vi "Pega_Tags_cluster_entrada.vi"() -> (1 "TipoVariavel":string[](array[string]), 2 "Array Tags":string[](array[string]))   [LabVIEW 2019]
uses:
  padrao_todos_os_dados_ENTRADA.ctl
  padrao_UCM.004.EEL.0300_ENTRADA.ctl
  padrao_UCM.004.EEL.0200_ENTRADA.ctl
  padrao_INTERNO.ctl
  padrao_ADAM_ENTRADA.ctl
panel:
  in  "todos_os_dados_ENTRADA":T1
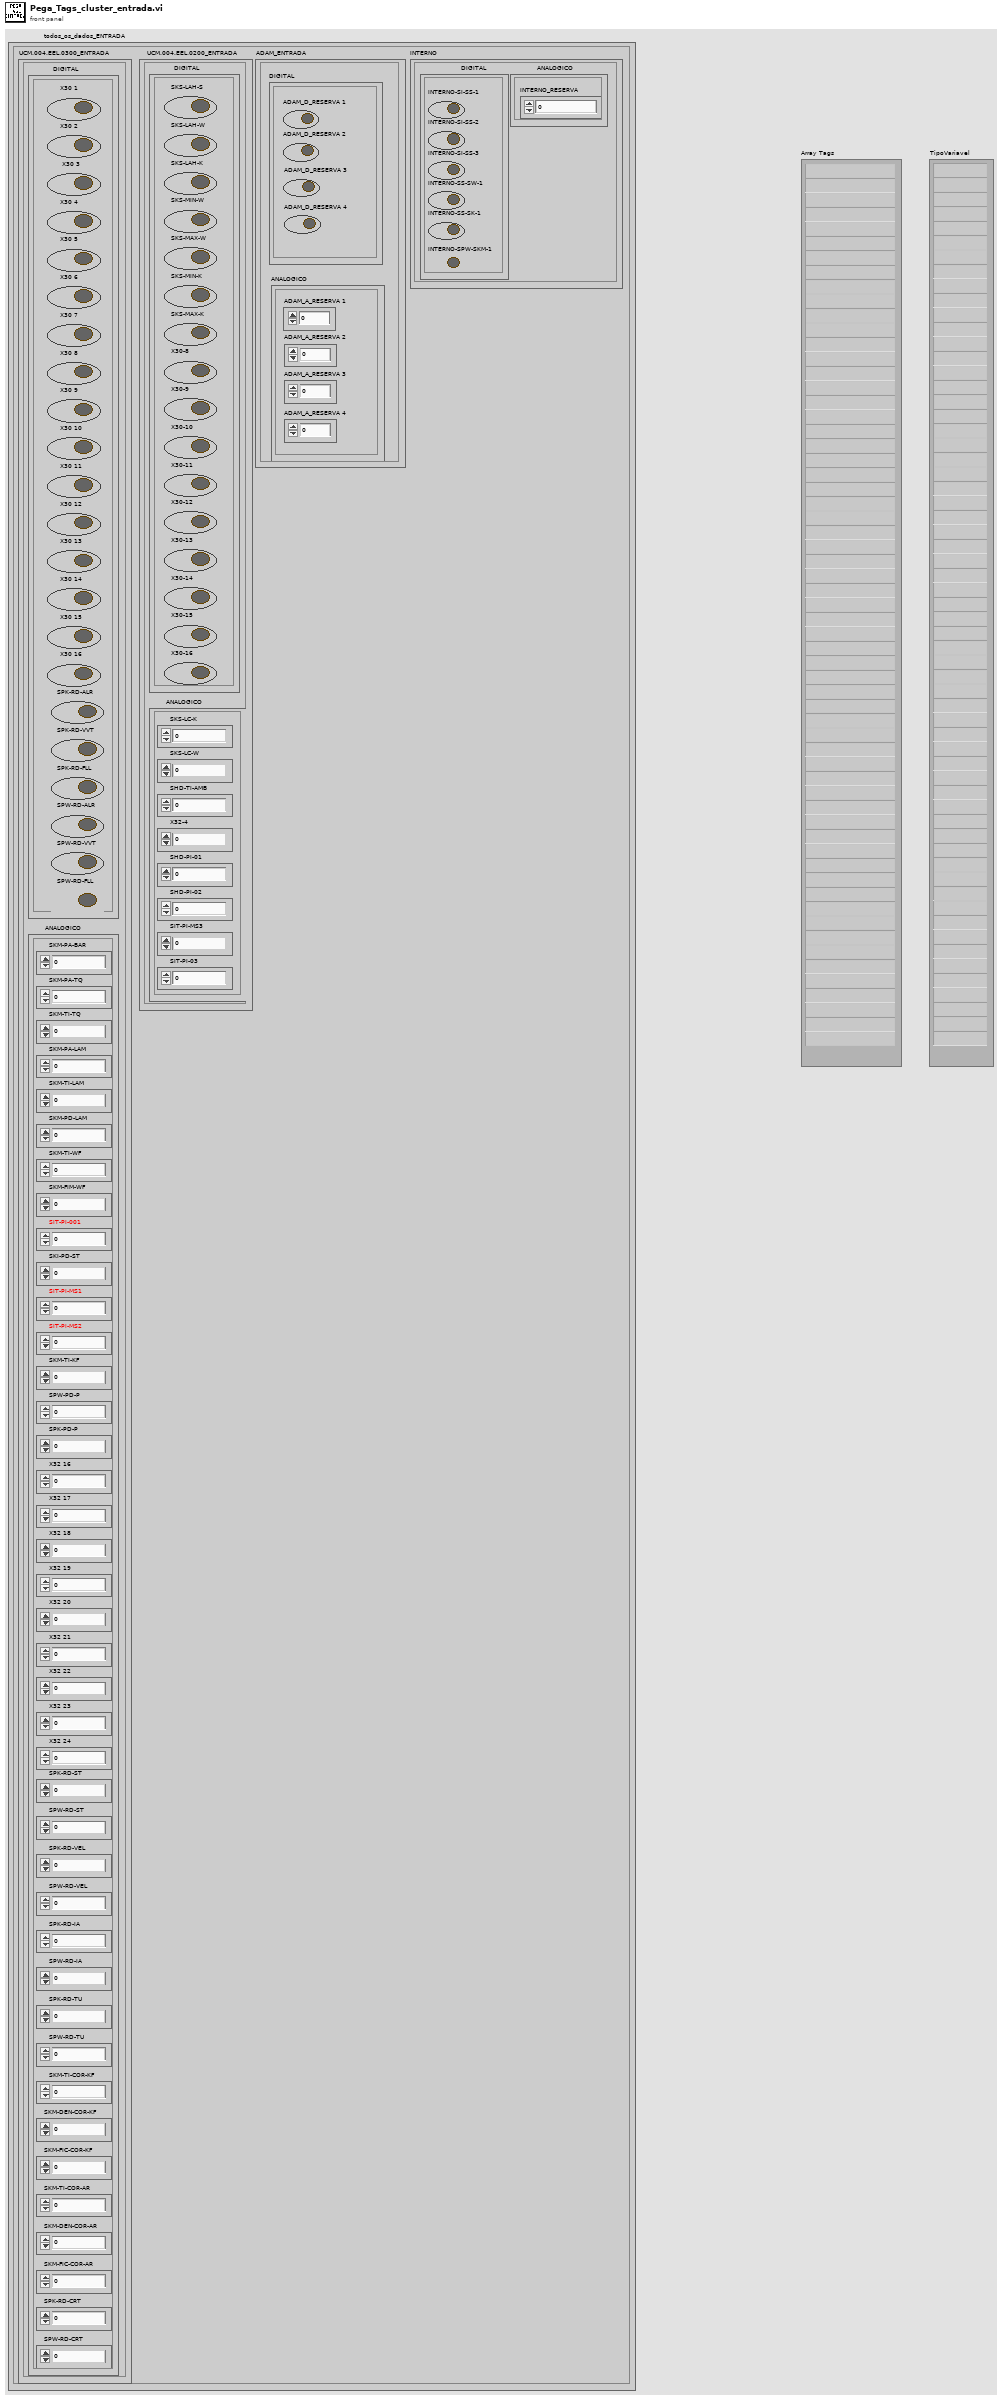
[diagram p1: front panel]
types:
  T1 = typedef "padrao_todos_os_dados_ENTRADA.ctl" = cluster{"UCM.004.EEL.0300_ENTRADA":T2, "UCM.004.EEL.0200_ENTRADA":T3, "INTERNO":T4, "ADAM_ENTRADA":T5}
  T2 = typedef "padrao_UCM.004.EEL.0300_ENTRADA.ctl" = cluster{"DIGITAL":cluster{"X30 1":bool, "X30 2":bool, "X30 3":bool, "X30 4":bool, "X30 5":bool, "X30 6":bool, "X30 7":bool, "X30 8":bool, "X30 9":bool, "X30 10":bool, "X30 11":bool, "X30 12":bool, "X30 13":bool, "X30 14":bool, "X30 15":bool, "X30 16":bool, "SPK-RD-ALR":bool, "SPK-RD-VVT":bool, "SPK-RD-FLL":bool, "SPW-RD-ALR":bool, "SPW-RD-VVT":bool, "SPW-RD-FLL":bool}, "ANALOGICO":cluster{"SKM-PA-BAR":i16, "SKM-PA-TQ":i16, "SKM-TI-TQ":i16, "SKM-PA-LAM":i16, "SKM-TI-LAM":i16, "SKM-PD-LAM":i16, "SKM-TI-WF":i16, "SKM-FIM-WF":i16, "SIT-PI-001":i16, "SKI-PD-ST":i16, "SIT-PI-MS1":i16, "SIT-PI-MS2":i16, "SKM-TI-KF":i16, "SPW-PD-P":i16, "SPK-PD-P":i16, "X32 16 ":i16, "X32 17":i16, "X32 18":i16, "X32 19":i16, "X32 20":i16, "X32 21":i16, "X32 22":i16, "X32 23":i16, "X32 24":i16, "SPK-RD-ST":i32, "SPW-RD-ST":i32, "SPK-RD-VEL":i32, "SPW-RD-VEL":i32, "SPK-RD-IA":i32, "SPW-RD-IA":i32, "SPK-RD-TU":i32, "SPW-RD-TU":i32, "SKM-TI-COR-KF":dbl, "SKM-DEN-COR-KF":dbl, "SKM-FIC-COR-KF":dbl, "SKM-TI-COR-AR":dbl, "SKM-DEN-COR-AR":dbl, "SPK-RD-CRT":dbl, "SPW-RD-CRT":dbl, "SKM-FIC-COR-AR":dbl}}
  T3 = typedef "padrao_UCM.004.EEL.0200_ENTRADA.ctl" = cluster{"DIGITAL":cluster{"SKS-LAH-S":bool, "SKS-LAH-W":bool, "SKS-LAH-K":bool, "SKS-MIN-W":bool, "SKS-MAX-W":bool, "SKS-MIN-K":bool, "SKS-MAX-K":bool, "X30-8":bool, "X30-9":bool, "X30-10":bool, "X30-11":bool, "X30-12":bool, "X30-13":bool, "X30-14":bool, "X30-15":bool, "X30-16":bool}, "ANALOGICO":cluster{"SKS-LC-K":i16, "SKS-LC-W":i16, "SHD-TI-AMB":i16, "X32-4":i16, "SHD-PI-01":i16, "SHD-PI-02":i16, "SIT-PI-MS3":i16, "SIT-PI-03":i16}}
  T4 = typedef "padrao_INTERNO.ctl" = cluster{"DIGITAL":cluster{"INTERNO-SI-SS-1":bool, "INTERNO-SI-SS-2":bool, "INTERNO-SI-SS-3":bool, "INTERNO-SS-SW-1":bool, "INTERNO-SS-SK-1":bool, "INTERNO-SPW-SKM-1":bool}, "ANALOGICO":cluster{"INTERNO_RESERVA":dbl}}
  T5 = typedef "padrao_ADAM_ENTRADA.ctl" = cluster{"DIGITAL":cluster{"ADAM_D_RESERVA 1":bool, "ADAM_D_RESERVA 2":bool, "ADAM_D_RESERVA 3":bool, "ADAM_D_RESERVA 4":bool}, "ANALOGICO":cluster{"ADAM_A_RESERVA 1":dbl, "ADAM_A_RESERVA 2":dbl, "ADAM_A_RESERVA 3":dbl, "ADAM_A_RESERVA 4":dbl}}
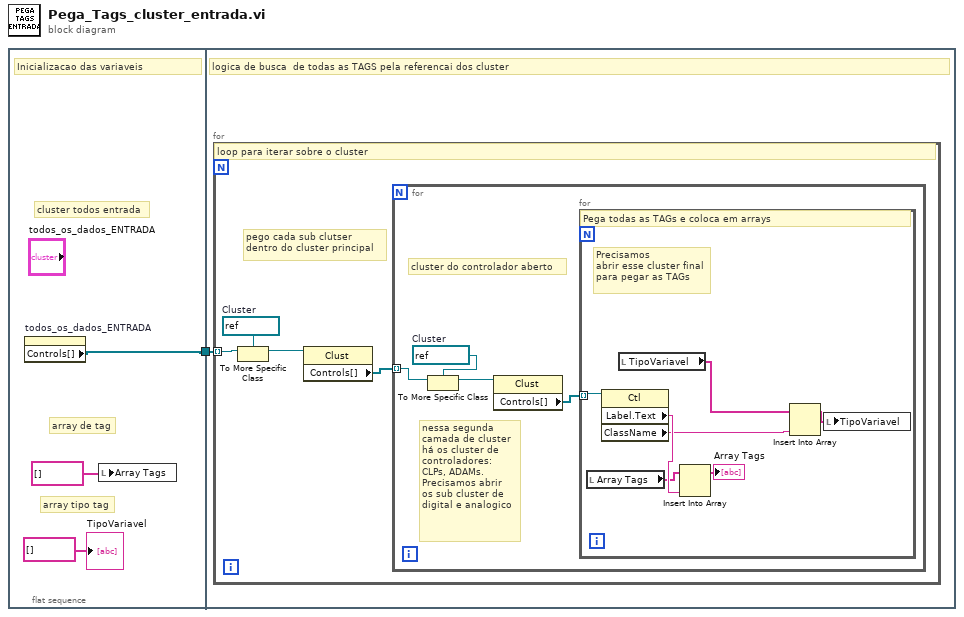
[diagram p0: block diagram]
diagram:
  n1 = flat-sequence {
    tunnel: [w2] -> w1
    tunnel: w1 -> [w5]
    frame #0 {
      # "cluster todos entrada"
      # "array tipo tag"
      # "array de tag"
      # "Inicializacao das variaveis"
      n2 = property on="todos_os_dados_ENTRADA" class="Clust (strict)"() -> ("Controls[]"=w2:refnum<vi>[])  [unwired: 2 in, 2 out]
      n3 = local write "Array Tags"(string[] [] ("Array")) -> ()
      "TipoVariavel" <- string[] [] ("Array")
    }
    frame #1 {
      # "logica de busca  de todas as TAGS pela referencai dos cluster"
      n4 = for {
        tunnel: w5 -> [w6] mode=indexing
        w9 = refnum<vi> refnum  # Cluster
        # "pego cada sub clutser \ndentro do cluster principal"
        # "loop para iterar sobre o cluster"
        n5 = To More Specific Class(target class=w9, reference=w6) -> (specific class reference=w7:refnum<vi>)  [unwired: 1 in, 1 out]
        n6 = property on="Property Node" class="Clust"(reference=w7) -> ("Controls[]"=w8:refnum<vi>[])  [unwired: 1 in, 2 out]
        n7 = for {
          tunnel: w8 -> [w12] mode=indexing
          w11 = refnum<vi> refnum  # Cluster
          # "nessa segunda \ncamada de cluster\nhá os cluster de \ncontroladores:\nCLPs, ADAMs.\nPrecisamos abrir \nos sub cluster de\ndigital e analogico"
          # "cluster do controlador aberto"
          n8 = To More Specific Class(target class=w11, reference=w12) -> (specific class reference=w13:refnum<vi>)  [unwired: 1 in, 1 out]
          n9 = property on="Property Node" class="Clust"(reference=w13) -> ("Controls[]"=w10:refnum<vi>[])  [unwired: 1 in, 2 out]
          n10 = for {
            tunnel: w10 -> [w20] mode=indexing
            # "Precisamos\nabrir esse cluster final\npara pegar as TAGs"
            # "Pega todas as TAGs e coloca em arrays"
            n11 = local read "Array Tags"() -> (w17:string[])
            n12 = property class="Ctl"(reference=w20) -> ("Label.Text"=w19:string, "ClassName"=w15:string)  [unwired: 1 in, 2 out]
            n13 = local read "TipoVariavel"() -> (w16:string[])
            n14 = Insert Into Array(array=w17, new element=w19) -> (→"Array Tags":string[])  [unwired: 1 in]
            n15 = Insert Into Array(array=w16, new element=w15) -> (w14:string[])  [unwired: 1 in]
            n16 = local write "TipoVariavel"(w14) -> ()
          }
        }
      }
    }
  }
